vi "Update Inventary.vi"(8 "error in (no error)":errorcluster, 9 "Indice":i32, 10 "Inventario":dbl, 11 "Soda Actor in":refnum<class "Soda Actor.lvclass">) -> (0 "error out":errorcluster, 3 "Soda Actor out":refnum<class "Soda Actor.lvclass">)   [LabVIEW 2020, in "Soda Actor.lvlib" / "Soda Actor.lvclass"]
uses:
  Soda Actor.lvclass
  Soda Actor.lvclass/Soda Actor.ctl
  <vilib>/Utility/config.llb/Write Key (String).vi
  <vilib>/Utility/config.llb/NI_LVConfig.lvlib
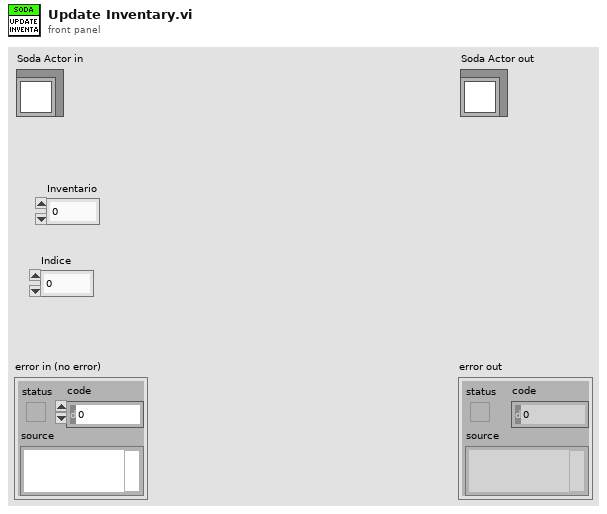
[diagram p1: front panel]
types:
  T1 = typedef "NI_LVConfig.lvlib/Config Data RefNum.ctl" = refnum<k1>
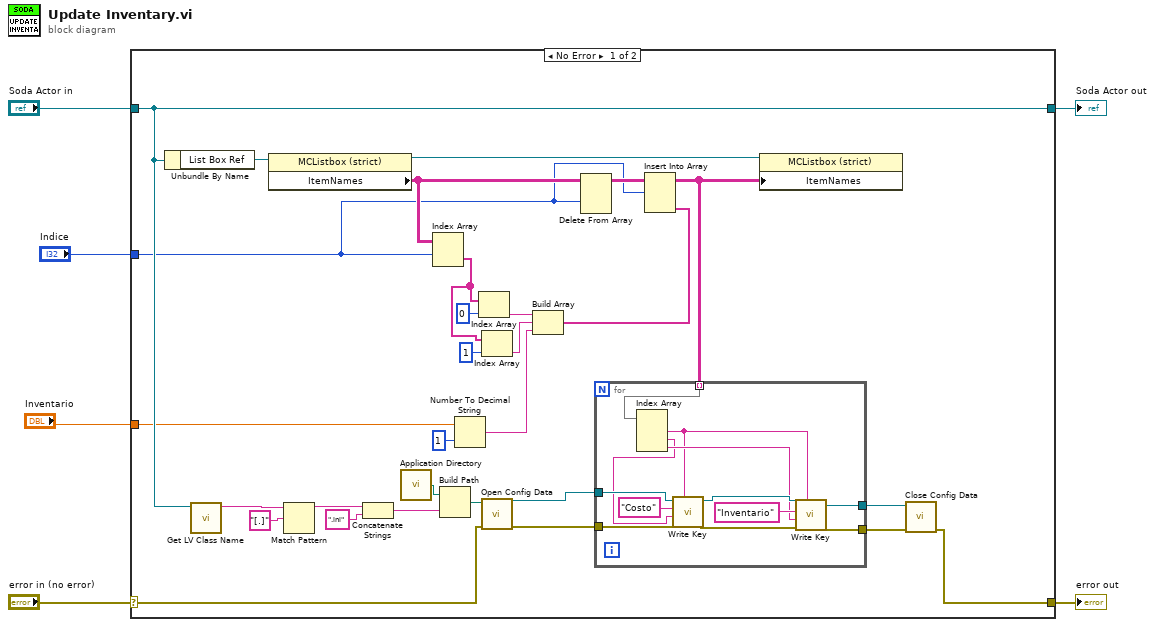
[diagram p0: block diagram]
diagram:
  n1 = case shown="No Error" "error in (no error)" {
    selector: "error in (no error)" -> [w8 w49]
    tunnel: [w7 w49] -> w5
    tunnel: [w34 w48] -> w3
    tunnel: "Soda Actor in" -> [w34 w48]
    tunnel: "Indice" -> [w12 _]
    tunnel: "Inventario" -> [w20 _]
    frame No Error {
      n2 = Unbundle By Name(w34) -> ("List Box Ref"=w35:refnum<vi>)
      n3 = call <vilib>:"Get LV Class Name.vi"("object"=w34) -> ("class name"=w27:string)  [unwired: 9 in, 1 out]
      n4 = property class="MCListbox (strict)"(reference=w35) -> (reference out=w9:refnum<vi>, "ItemNames"=w14:string[][])  [unwired: 1 in, 1 out]
      n5 = Match Pattern(string=w27, regular expression="[.]") -> (before substring=w28:string)  [unwired: 1 in, 3 out]
      n6 = Concatenate Strings(w28, ".ini") -> (w32:string)
      n7 = call <vilib>:"Application Directory.vi"() -> ("Application Directory"=w33:path)
      n8 = Index Array(array=w14, index (row)=w12) -> (element=w24:string[])  [unwired: 1 in]
      n9 = Build Path(base path=w33, name or relative path=w32) -> (appended path=w30:path)
      n10 = Number To Decimal String(number=w20, width (-)=i16 1) -> (decimal integer string=w21:string)
      n11 = Index Array(array=w24, index=0) -> (element=w23:string)
      n12 = Index Array(array=w24, index=1) -> (element=w22:string)
      n13 = call <vilib>:"Open Config Data.vi"("error in (no error)"=w8, "configuration file path"=w30) -> ("error out"=w17:errorcluster, "refnum"=w18:T1)  [unwired: 7 in, 1 out]
      n14 = Build Array(w23, w22, w21) -> (w11:string[])
      n15 = Delete From Array(array=w14, index (row)=w12) -> (array with subset deleted=w13:string[][])  [unwired: 2 in, 1 out]
      n16 = Insert Into Array(array=w13, index (row)=w12, new element=w11) -> (w10:string[][])  [unwired: 1 in]
      n17 = for {
        tunnel: w18 -> [w45]
        tunnel: w17 -> [w44]
        tunnel: [w41] -> w16
        tunnel: [w40] -> w15
        tunnel: w10 -> [w39] mode=indexing
        n18 = Index Array(array=w39) -> (element #1=w37:string, element #2=w36:string, element #3=w38:string)  [unwired: 3 in]
        n19 = call-poly <vilib>:"Write Key.vi"("section"=w37, "error in (no error)"=w44, "value"=w36, "key"="Costo", "refnum"=w45) -> ("error out"=w42:errorcluster, "refnum out"=w43:T1)  [unwired: 4 in, 1 out]
        n20 = call-poly <vilib>:"Write Key.vi"("section"=w37, "error in (no error)"=w42, "value"=w38, "key"="Inventario", "refnum"=w43) -> ("error out"=w40:errorcluster, "refnum out"=w41:T1)  [unwired: 4 in, 1 out]
      }
      n21 = property class="MCListbox (strict)"(reference=w9, "ItemNames"=w10) -> ()  [unwired: 1 in, 2 out]
      n22 = call <vilib>:"Close Config Data.vi"("error in (no error)"=w15, "refnum"=w16) -> ("error out"=w7:errorcluster)  [unwired: 8 in, 1 out]
    }
    frame Error {
    }
  }
  "error out" <- w5
  "Soda Actor out" <- w3
